vi "RingArray and Ring.vi"(8 "ClusterInCluster":T1={"Cluster 3"={"Ring"=0, "ArrayRing"=[0, 0, 0, 0, 900]}} {"Cluster 3"."ArrayRing" items=["c"=0, "b"=900, "d"=10000, "a"=500]; "Cluster 3"."Ring" items=["c"=0, "b"=900, "d"=10000, "a"=500]}, 14 "Ring":i32(ring) items=["c"=0, "b"=900, "d"=10000, "a"=500], 17 "Array 3":cluster{"Ring":u16, "ArrayRing":i32[]}[](array[cluster]) {"ArrayRing" items=["c"=0, "b"=900, "d"=10000, "a"=500]; "Ring" items=["c"=0, "b"=900, "d"=10000, "a"=500]}, 20 "ArrayRing":i32[](array[ring])=[0, 0, 0, 0, 900, 10000] items=["c"=0, "b"=900, "d"=10000, "a"=500], 23 "Cluster 3":cluster{"Ring":u16, "ArrayRing":i64[]}={"Ring"=0, "ArrayRing"=[0, 0, 900, 0, 10000]} {"ArrayRing" items=["c"=0, "b"=900, "d"=10000, "a"=500]; "Ring" items=["c"=0, "b"=900, "d"=10000, "a"=500]}, 25 "Array 9":cluster{"Ring":u16, "ArrayRing":i16[]}[][](array[cluster])=[[{"Ring"=10000, "ArrayRing"=[10000]}], [{"Ring"=10000, "ArrayRing"=[0, 0, 0, 10000]}], [{"Ring"=0, "ArrayRing"=[]}], [{"Ring"=0, "ArrayRing"=[]}], [{"Ring"=0, "ArrayRing"=[]}], [{"Ring"=0, "ArrayRing"=[]}]] {"ArrayRing" items=["c"=0, "b"=900, "d"=10000, "a"=500]; "Ring" items=["c"=0, "b"=900, "d"=10000, "a"=500]}) -> (15 "Array 6":cluster{"Ring":u16, "ArrayRing":u16[]}[](array[cluster]) {"ArrayRing" items=["c"=0, "b"=900, "d"=10000, "a"=500]; "Ring" items=["c"=0, "b"=900, "d"=10000, "a"=500]}, 16 "Ring 2":u16(ring) items=["c"=0, "b"=900, "d"=10000, "a"=500], 21 "ArrayRing 2":u16[](array[ring]) items=["c"=0, "b"=900, "d"=10000, "a"=500], 24 "Cluster 6":cluster{"Ring":u16, "ArrayRing":u16[]} {"ArrayRing" items=["c"=0, "b"=900, "d"=10000, "a"=500]; "Ring" items=["c"=0, "b"=900, "d"=10000, "a"=500]}, 27 "Array 10":cluster{"Ring":u16, "ArrayRing":u16[]}[][](array[cluster]) {"ArrayRing" items=["c"=0, "b"=900, "d"=10000, "a"=500]; "Ring" items=["c"=0, "b"=900, "d"=10000, "a"=500]})   [LabVIEW 2012]
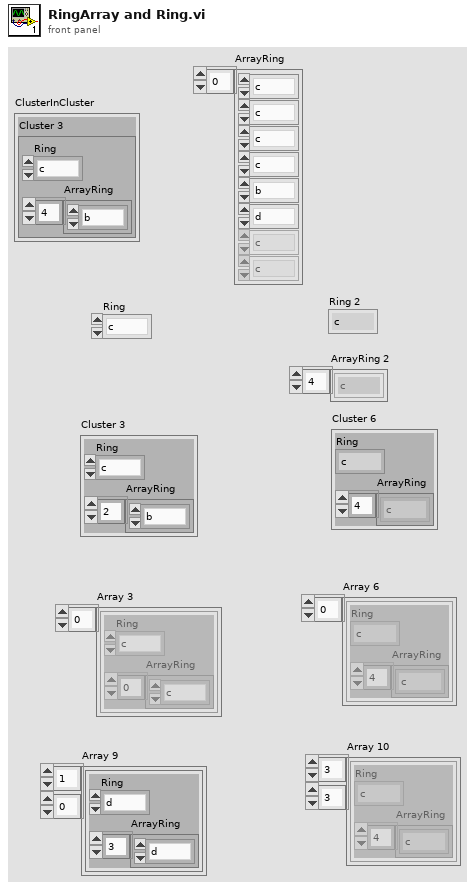
[diagram p1: front panel]
types:
  T1 = cluster{"Cluster 3":cluster{"Ring":u16, "ArrayRing":i64[]}}
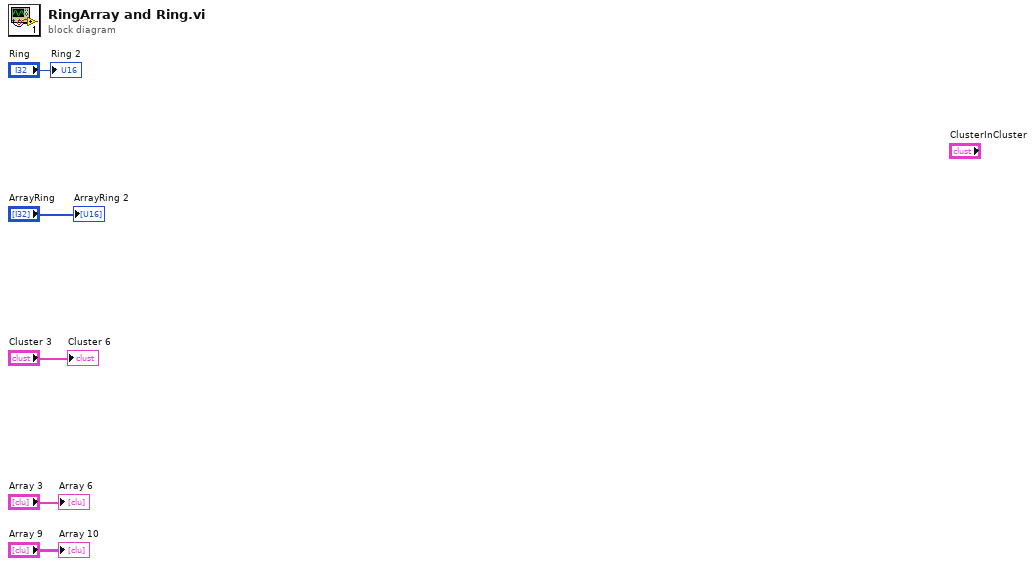
[diagram p0: block diagram]
diagram:
  "Ring 2" <- "Ring"
  "ArrayRing 2" <- "ArrayRing"
  "Cluster 6" <- "Cluster 3"
  "Array 6" <- "Array 3"
  "Array 10" <- "Array 9"
